vi "Get Custom Device Name.vi"(8 "error in":errorcluster, 11 "ni-switch custom device in":T1 format="%.0x") -> (0 "error out":errorcluster, 2 "name":string, 3 "ni-switch custom device out":T1 format="%.0x")   [LabVIEW 2020, in "NI-SWITCH Scripting.lvlib"]
uses:
  NI-SWITCH Scripting.lvlib
  <vilib>/NI VeriStand/Custom Device API/Custom Device Item Ref.ctl
  <vilib>/NI VeriStand/Custom Device API/Custom Device API.lvlib
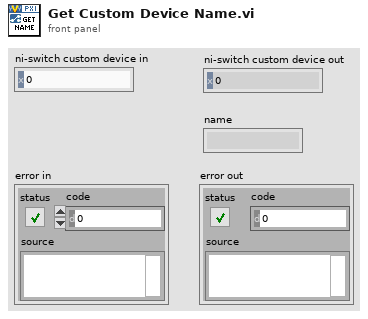
[diagram p1: front panel]
types:
  T1 = typedef "Custom Device API.lvlib/Custom Device Item Ref.ctl" = u64
  T2 = typedef "Custom Device API.lvlib/Custom Device Item Info.ctl" = cluster{"Name":string, "Is Channel":bool, "GUID":string, "Is Waveform":bool}
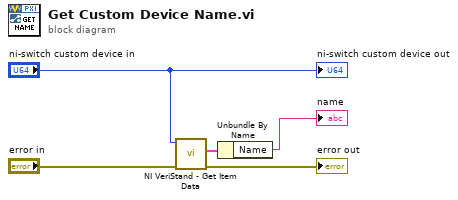
[diagram p0: block diagram]
diagram:
  n1 = call <vilib>:"NI VeriStand - Get Item Data.vi"("error in (no error)"="error in", "Item Ref in"="ni-switch custom device in") -> ("error out"=→"error out":errorcluster, "Item Info"=w5:T2)  [unwired: 6 in, 2 out]
  n2 = Unbundle By Name(w5) -> ("Name"=→"name":string)
  "ni-switch custom device out" <- "ni-switch custom device in"
